vi "Sim Scout_velocity.vi"() -> ()   [LabVIEW 2019]
uses:
  Patrolrobot/Ctrl/agv_cmd_v.ctl
panel:
  out "Velocity Graph":cluster{"X":dbl, "Y":dbl}[](graph)
  in  "stop":bool
  in  "deg gap":dbl(slide) scale=-30.0..30.0
  in  "linear v":dbl
  in  "decrease factor":dbl
  out "velocity_out":dbl
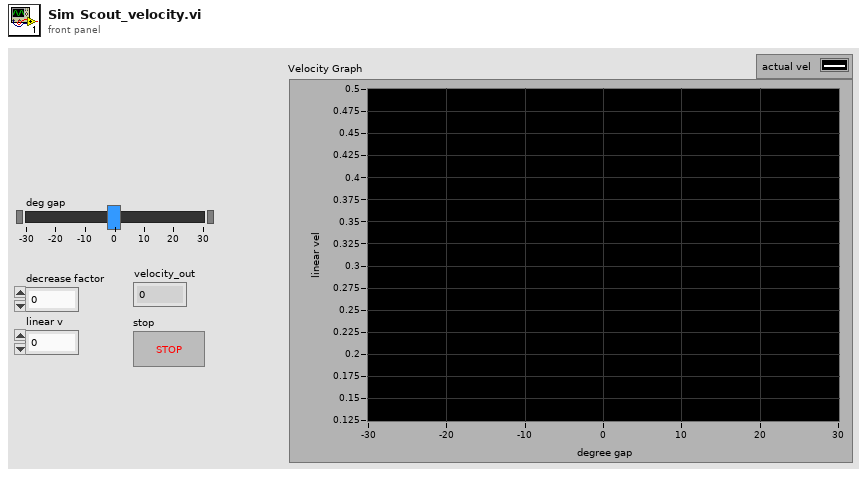
[diagram p1: front panel]
types:
  T1 = typedef "agv_cmd_v.ctl" = enum16{"write limit", "init stop", "write", "read"}
  T2 = cluster{"limit_linear-v":dbl, "limit_angular-v":dbl}
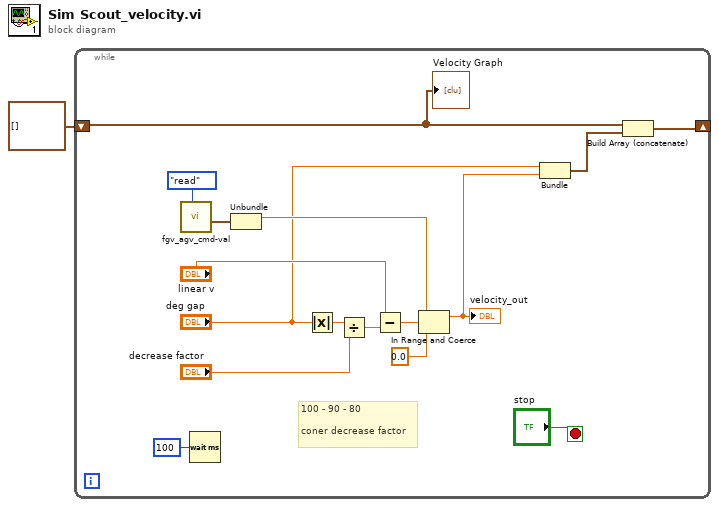
[diagram p0: block diagram]
diagram:
  n1 = while {
    shift-right: [w6] -> _
    shift-left: cluster{"limit_linear-v":dbl, "deg gap":dbl}[] [] -> [w4]
    stop <- "stop" stop-if-true
    # "100 - 90 - 80\n\nconer decrease factor"
    n2 = call "fgv_agv_cmd-val.vi"("cmd"=agv_cmd_v."read") -> ("limits out"=w15:T2)  [unwired: 9 in, 1 out]
    n3 = Wait (ms)(milliseconds to wait=u32 100) -> ()  [unwired: 1 out]
    n4 = Unbundle(w15) -> ("limit_linear-v"=w14:dbl)  [unwired: 1 out]
    n5 = Absolute Value(x="deg gap") -> (abs(x)=w11:dbl)
    n6 = Divide(x=w11, y="decrease factor") -> (x/y=w13:dbl)
    n7 = Subtract(x="linear v", y=w13) -> (x-y=w12:dbl)
    n8 = In Range and Coerce(upper limit=w14, x=w12, lower limit=0.0 ("하위 리미트")) -> (coerced(x)=w2:dbl)  [unwired: 1 out]
    "velocity_out" <- w2
    n9 = Bundle("deg gap"="deg gap", "limit_linear-v"=w2) -> (w5:cluster{"deg gap":dbl, "limit_linear-v":dbl})  [unwired: 1 in]
    n10 = Build Array (concatenate)(w4, w5) -> (w6:cluster{"deg gap":dbl, "limit_linear-v":dbl}[])
    "Velocity Graph" <- w4
  }
